vi "DefineSpectrumSFAT.vi"(8 "error in":errorcluster, 10 "SFAT Settings":T2, 11 "connection ID in":refnum<k5>) -> (0 "error out":errorcluster, 1 "Error Info":T1, 2 "OK":bool, 3 "connection ID out":refnum<k5>, 4 "Log String":string)   [LabVIEW 2020, in "ProdigyRemoteControl.lvlib"]
uses:
  ProdigyRemoteControl.lvlib
  DEFINITIONS/DEF_SFAT_Settings.ctl
  DEFINITIONS/DEF_RcError.ctl
  DEFINITIONS/DEF_RcCmd.ctl
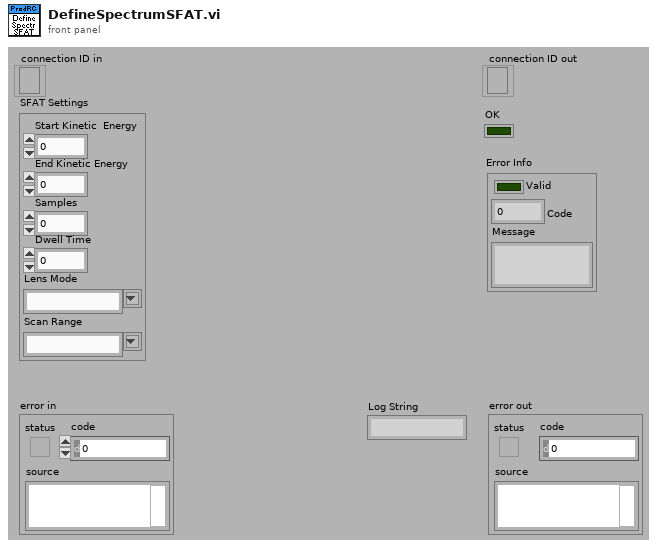
[diagram p1: front panel]
types:
  T1 = typedef "ProdigyRemoteControl.lvlib/DEF_RcError.ctl" = cluster{"Valid":bool, "Code":u16, "Message":string}
  T2 = typedef "ProdigyRemoteControl.lvlib/DEF_SFAT_Settings.ctl" = cluster{"Start Kinetic  Energy":dbl, "End Kinetic Energy":dbl, "Samples":u32, "Dwell Time":dbl, "Scan Range":string, "Lens Mode":string}
  T3 = typedef "ProdigyRemoteControl.lvlib/DEF_RcCmd.ctl" = string
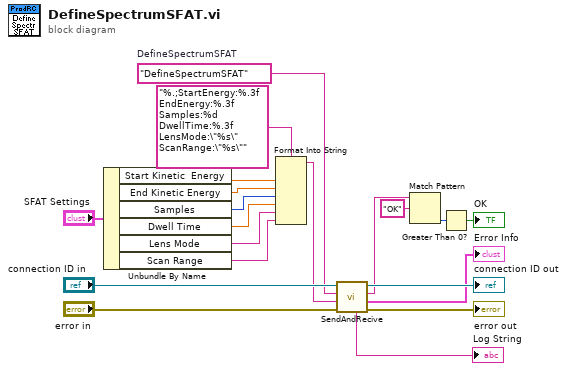
[diagram p0: block diagram]
diagram:
  w15 = T3 "DefineSpectrumSFAT"  # DefineSpectrumSFAT
  n1 = Unbundle By Name("SFAT Settings") -> ("Start Kinetic  Energy"=w13:dbl, "End Kinetic Energy"=w12:dbl, "Samples"=w11:u32, "Dwell Time"=w10:dbl, "Lens Mode"=w9:string, "Scan Range"=w8:string)
  n2 = Format Into String(format string="%.;StartEnergy:%.3f EndEnergy:%.3f Samples:%d DwellTime:%.3f LensMode:\"%s\" ScanRange:\"%s\"", w13, w12, w11, w10, w9, w8) -> (resulting string=w7:string)  [unwired: 2 in, 1 out]
  n3 = call "SendAndRecive.vi"("error in"="error in", "Parameters"=w7, "Command"=w15, "connection ID in"="connection ID in") -> ("error out"=→"error out":errorcluster, "Error Info"=→"Error Info":T1, "Answer"=w2:string, "connection ID out"=→"connection ID out":refnum<k5>, "Log String"=→"Log String":string)  [unwired: 3 in]
  n4 = Match Pattern(string=w2, regular expression="OK") -> (offset past match=w4:i32)  [unwired: 1 in, 3 out]
  n5 = Greater Than 0?(x=w4) -> (x > 0?=→"OK":bool)
